vi "Fit Model to Plot v3.vi"(0 "Fit Plot Information":T8={"XY Graph Ref"=refnum, "Mouse Coordinates"={"X"=0.0, "Y"=0.0}, "Fit Model"=enum."Select a Fit Model...", "Plot Index"=-1}, 5 "Fit Settings":T2={"Use Original Plot # Points"=TRUE, "# Fit Plot Points"=0, "Fitting Method"=0, "Weighted Fit"=TRUE, "Show All Fit Components"=FALSE, "Axis Type"=0, "Show Fit Residuals"=TRUE, "Residual Type"=enum."Standard", "Fitting Algorithm"=enum."Levenberg-Marquardt"} {"Axis Type" items=["Linear", "Logarithmic"]; "Fitting Method" items=["Least Square", "Least Absolute Residual", "Bisquare"]}, 7 "Additional Parameters (in)":variant, 9 "Fixed Parameters":T7, 11 "error in (no error)":errorcluster, 12 "Termination Criteria":T1={"Max Iterations"=1000, "Max Function Calls"=10000, "Max Time"=1000.0, "Function Tolerance"=1e-06, "Parameter Tolerance"=1e-06, "Gradient Tolerance"=1e-06, "Min Lambda"=1e-06, "Max Lambda"=1000000.0, "Initial Tick Count"=0}, 13 "Send Graph to Notebook? (F)":bool) -> (1 "Fitted Plot":cluster{"X Array":dbl[], "Y Array":dbl[]}, 2 "Graph Name":string, 3 "Plot Name":string, 4 "Best Fit":dbl[](array[numeric]), 6 "Fit Parameter Names":string[](array[string]), 8 "Additional Parameters (out)":variant, 10 "Fit Parameter Values":dbl[](array[numeric]), 14 "Fit Result String":string, 15 "error out":errorcluster)   [LabVIEW 2019]
uses:
  Fit Plot Request Information.ctl
  <vilib>/Utility/miscctls.llb/LVPointDoubleTypeDef.ctl
  Fit Models.ctl
  D-Only Fixed Parameters.ctl
  Fit Settings.ctl
  <vilib>/Analysis/6fits.llb/Curve Fitting Criteria.ctl
  Calc/Ramp Type.ctl
  Residual Type.ctl
  Non-linear Fitting Algorithm.ctl
  My Fit Stopping Criteria.ctl
  Graphs/XY Graph/XY Graph Add-Ons.lvlib
  <vilib>/Analysis/NI_AALPro.lvlib
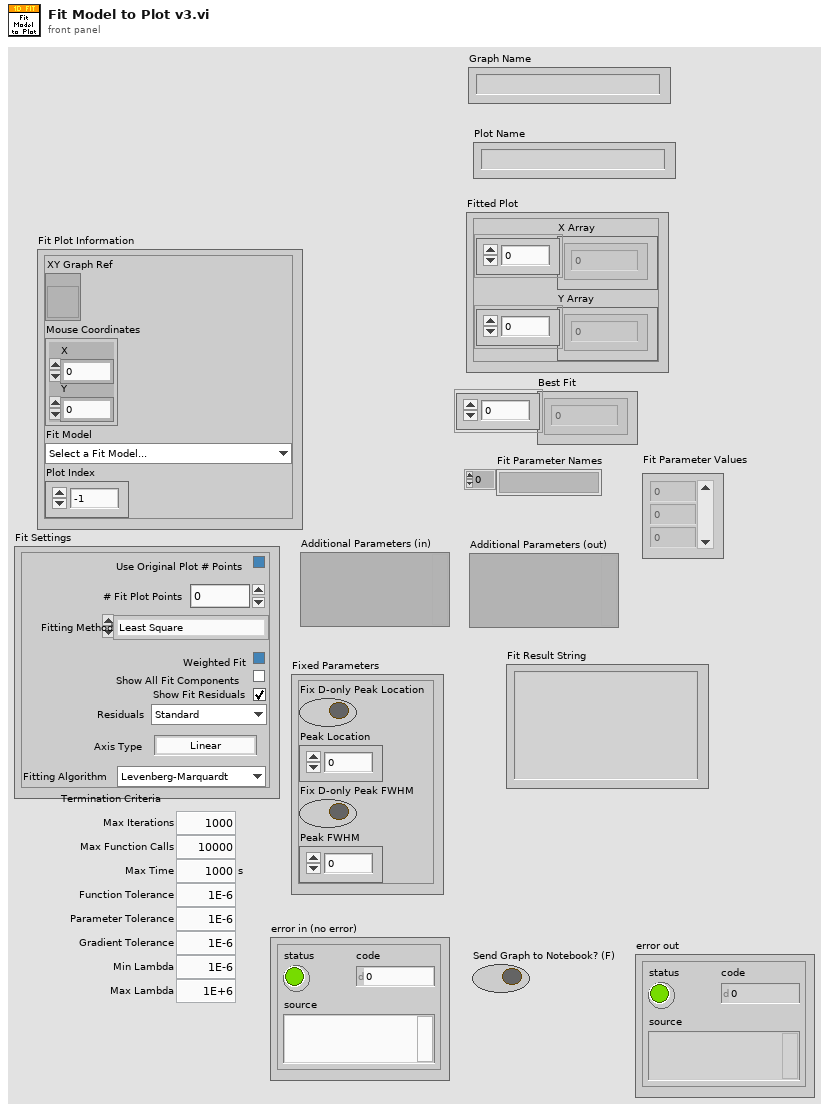
[diagram p1: front panel]
types:
  T1 = typedef "My Fit Stopping Criteria.ctl" = cluster{"Max Iterations":i32, "Max Function Calls":i32, "Max Time":dbl[unit], "Function Tolerance":dbl, "Parameter Tolerance":dbl, "Gradient Tolerance":dbl, "Min Lambda":dbl, "Max Lambda":dbl, "Initial Tick Count":u32}
  T2 = typedef "Fit Settings.ctl" = cluster{"Use Original Plot # Points":bool, "# Fit Plot Points":u32, "Fitting Method":T3, "Weighted Fit":bool, "Show All Fit Components":bool, "Axis Type":T4, "Show Fit Residuals":bool, "Residual Type":T5, "Fitting Algorithm":T6}
  T3 = typedef "NI_AALPro.lvlib/Curve Fitting Criteria.ctl" = u16
  T4 = typedef "Ramp Type.ctl" = u16
  T5 = typedef "Residual Type.ctl" = enum16{"Standard", "Normalized", "Reduced"}
  T6 = typedef "Non-linear Fitting Algorithm.ctl" = enum16{"Levenberg-Marquardt", "Trust-Region Dogleg"}
  T7 = typedef "D-Only Fixed Parameters.ctl" = cluster{"Fix D-only Peak Location":bool, "Peak Location":dbl, "Fix D-only Peak FWHM":bool, "Peak FWHM":dbl}
  T8 = typedef "Fit Plot Request Information.ctl" = cluster{"XY Graph Ref":refnum<vi>, "Mouse Coordinates":T9, "Fit Model":T10, "Plot Index":i32}
  T9 = typedef "LVPointDoubleTypeDef.ctl" = cluster{"X":dbl, "Y":dbl}
  T10 = typedef "Fit Models.ctl" = enum16{"Select a Fit Model...", "           Single Peak", "Gaussian", "Asymmetric Gaussian", "Lorentzian", "Asymmetric Lorentzian", "Gaussian/Lorentzian", "Lorentzian/Gaussian", "           Double Peak", "Two Gaussians", "Two Asymmetric Gaussians", "Two H-Connected Gaussians", "Two T-Connected Gaussians", "Two H-Connected Asymmetric Gaussians", "Two T-Connected Asymmetric Gaussians", "           Triple Peak", "Three Gaussians", "Three Asymmetric Gaussians", "              Decays", "1-Exponential", "IRF*PSED", "2-Exponentials", "               ACF", "2D Gaussian ACF", "2D Gaussian + Blinking ACF", "2D Gaussian + Flow ACF", "3D Gaussian ACF", "3D Gaussian + Blinking ACF", "             Multiplot", "2D Gaussian ACF & 2D Gaussian + Flow ACF"}
  T11 = typedef "XY Graph Add-Ons.lvlib/XY Graph Refnum.ctl" = refnum<vi>
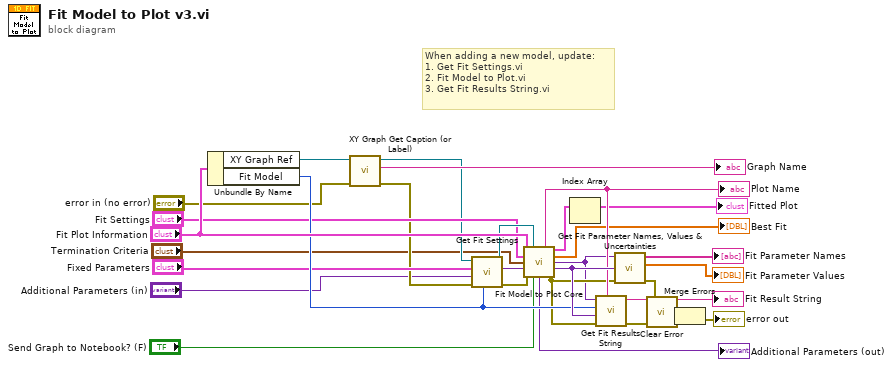
[diagram p0: block diagram]
diagram:
  # "When adding a new model, update:\n1. Get Fit Settings.vi\n2. Fit Model to Plot.vi\n3. Get Fit Results String.vi"
  n1 = Unbundle By Name("Fit Plot Information") -> ("XY Graph Ref"=w12:refnum<vi>, "Fit Model"=w21:T10)
  n2 = call "XY Graph Get Caption (or Label).vi"("error in (no error)"="error in (no error)", "XYGraph in"=w12) -> ("error out"=w8:errorcluster, "Caption (or Label) Text"=→"Graph Name":string, "XYGraph out"=w9:T11)  [unwired: 7 in]
  n3 = call "Get Fit Settings.vi"("Fit Model"=w21, "Error In"=w8, "Additional Parameters"="Additional Parameters (in)", "Fixed Parameters"="Fixed Parameters", "XY Graph Ref"=w9) -> ("Error Out"=w17:errorcluster, "Additional Fit Settings"=w20:variant, "LM Function & Gradient"=w24:refnum<vi>)  [unwired: 4 in]
  n4 = call "Fit Model to Plot Core.vi"("Fit Plot Information"="Fit Plot Information", "LM Function & Gradient"=w24, "Fit Settings"="Fit Settings", "Termination Criteria"="Termination Criteria", "Additional Data (in)"=w20, "error in (no error)"=w17, "Send Graph to Notebook?"="Send Graph to Notebook? (F)") -> ("Plot Name"=w23:string, "Array of Plots (Fit, Components, Residuals)"=w26:cluster{"X Array":dbl[], "Y Array":dbl[]}[], "best nonlinear fit"=→"Best Fit":dbl[], "Fit Parameters Cluster"=w4:variant, "Fit Parameters Uncertainties Cluster"=w25:variant, "Additional Data (out)"=→"Additional Parameters (out)":variant, "error out"=w16:errorcluster)  [unwired: 1 in, 1 out]
  "Plot Name" <- w23
  n5 = Index Array(array=w26) -> (element=→"Fitted Plot":cluster{"X Array":dbl[], "Y Array":dbl[]})  [unwired: 1 in]
  n6 = call "Get Fit Results String.vi"("Plot Name"=w23, "error in (no error)"=w16, "Fit Parameters Uncertainties Cluster"=w25, "Fit Model"=w21, "Fit Parameters Cluster"=w4) -> ("error out"=w14:errorcluster, "Fit Results String"=→"Fit Result String":string)  [unwired: 5 in]
  n7 = call "Get Fit Parameter Names, Values & Uncertainties.vi"("error in (no error)"=w16, "Fit Parameter Uncertainties"=w25, "Fit Parameters"=w4) -> ("Error Out"=w22:errorcluster, "Fit Parameter Values"=→"Fit Parameter Values":dbl[], "Fit Parameter Names"=→"Fit Parameter Names":string[])  [unwired: 5 in, 1 out]
  n8 = call "Clear Error.vi"("Error In"=w22) -> ("no Error Out"=w13:errorcluster)  [unwired: 8 in]
  n9 = Merge Errors(w13, w14) -> (→"error out":errorcluster)
